vi "BoardUpdate.vi"(1 "Array":i32[][](array[numeric])=[[-3, -5, -4, -2, -1, -4, -5, -3], [-6, -6, -6, -6, -6, -6, -6, -6], [0, 0, 0, 0, 0, 0, 0, 0], [0, 0, 0, 0, 0, 0, 0, 0], [0, 0, 0, 0, 0, 0, 0, 0], [0, 0, 0, 0, 0, 0, 0, 0], [6, 6, 6, 6, 6, 6, 6, 6], [3, 5, 4, 2, 1, 4, 5, 3]], 2 "Clust Refnum":refnum<vi>) -> ()   [LabVIEW 2014]
doc: "Initialize cluster without array input, or update cluster with array input."
panel:
  in  "Colors [4]":cluster{u32, u32}[](array[cluster])=[{12369084, 12369084}, {9868950, 9868950}, {12369084, 12369084}, {9868950, 9868950}]
  out "Board 2":T1
  in  "Board":T1
  # "1:King\n2:Queen\n3:Rook\n4:Bishop\n5:Knight\n6:Pawn"
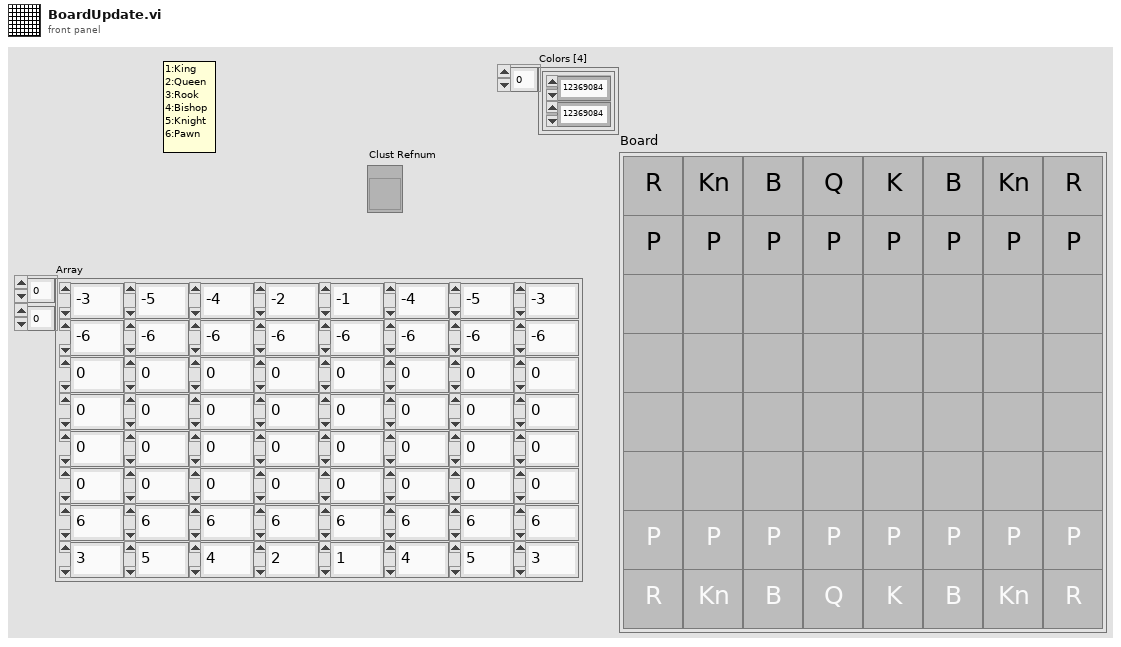
[diagram p1: front panel]
types:
  T1 = cluster{"OK Button 01":bool, "OK Button 02":bool, "OK Button 03":bool, "OK Button 04":bool, "OK Button 05":bool, "OK Button 06":bool, "OK Button 07":bool, "OK Button 08":bool, "OK Button 09":bool, "OK Button 10":bool, "OK Button 11":bool, "OK Button 12":bool, "OK Button 13":bool, "OK Button 14":bool, "OK Button 15":bool, "OK Button 16":bool, "OK Button 17":bool, "OK Button 18":bool, "OK Button 19":bool, "OK Button 20":bool, "OK Button 21":bool, "OK Button 22":bool, "OK Button 23":bool, "OK Button 24":bool, "OK Button 25":bool, "OK Button 26":bool, "OK Button 27":bool, "OK Button 28":bool, "OK Button 29":bool, "OK Button 30":bool, "OK Button 31":bool, "OK Button 32":bool, "OK Button 33":bool, "OK Button 34":bool, "OK Button 35":bool, "OK Button 36":bool, "OK Button 37":bool, "OK Button 38":bool, "OK Button 39":bool, "OK Button 40":bool, "OK Button 41":bool, "OK Button 42":bool, "OK Button 43":bool, "OK Button 44":bool, "OK Button 45":bool, "OK Button 46":bool, "OK Button 47":bool, "OK Button 48":bool, "OK Button 49":bool, "OK Button 50":bool, "OK Button 51":bool, "OK Button 52":bool, "OK Button 53":bool, "OK Button 54":bool, "OK Button 55":bool, "OK Button 56":bool, "OK Button 57":bool, "OK Button 58":bool, "OK Button 59":bool, "OK Button 60":bool, "OK Button 61":bool, "OK Button 62":bool, "OK Button 63":bool, "OK Button 64":bool}
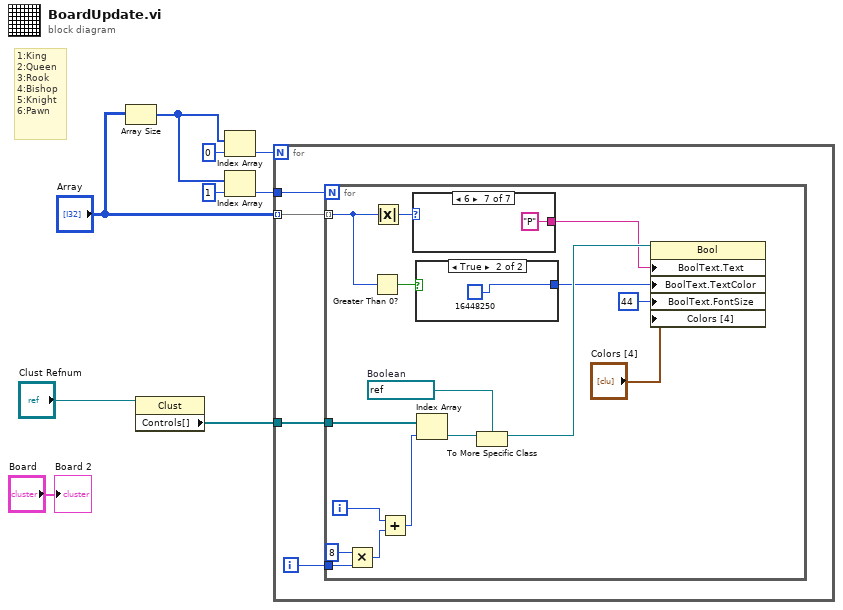
[diagram p0: block diagram]
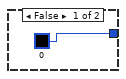
[diagram p2: hidden frame]
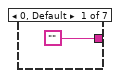
[diagram p3: hidden frame]
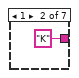
[diagram p4: hidden frame]
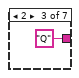
[diagram p5: hidden frame]
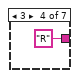
[diagram p6: hidden frame]
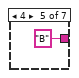
[diagram p7: hidden frame]
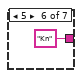
[diagram p8: hidden frame]
diagram:
  # "1:King\n2:Queen\n3:Rook\n4:Bishop\n5:Knight\n6:Pawn"
  n1 = Array Size(array="Array") -> (size(s)=w5:i32[])
  n2 = property class="Clust"(reference="Clust Refnum") -> ("Controls[]"=w3:refnum<vi>[])  [unwired: 1 in, 2 out]
  n3 = Index Array(array=w5, index=0) -> (element=w8:i32)
  n4 = Index Array(array=w5, index=1) -> (element=w4:i32)
  n5 = for {
    N: w8 -> [_]
    tunnel: "Array" -> [w12] mode=indexing
    tunnel: w4 -> [w13]
    tunnel: w3 -> [w11]
    i -> [w10]
    n6 = for {
      N: w13 -> [_]
      tunnel: w12 -> [w18] mode=indexing
      tunnel: w11 -> [w25]
      tunnel: w10 -> [w29]
      i -> [w27]
      w22 = refnum<vi> refnum  # Boolean
      n7 = Multiply(x=8, y=w29) -> (x*y=w26:i32)
      n8 = Greater Than 0?(x=w18) -> (x > 0?=w19:bool)
      n9 = Absolute Value(x=w18) -> (abs(x)=w20:i32)
      n10 = Add(x=w27, y=w26) -> (x+y=w24:i32)
      n11 = case shown="6" w20 {
        tunnel: ["" "K" "Q" "R" "B" "Kn" "P"] -> w16
        frame 0, Default {
        }
        frame 1 {
        }
        frame 2 {
        }
        frame 3 {
        }
        frame 4 {
        }
        frame 5 {
        }
        frame 6 {
        }
      }
      n12 = case shown="True" w19 {
        tunnel: [u32 0 u32 16448250] -> w17
        frame False {
        }
        frame True {
        }
      }
      n13 = Index Array(array=w25, index=w24) -> (element=w23:refnum<vi>)
      n14 = To More Specific Class(target class=w22, reference=w23) -> (specific class reference=w21:refnum<vi>)  [unwired: 1 in, 1 out]
      n15 = property class="Bool"(reference=w21, "BoolText.Text"=w16, "BoolText.TextColor"=w17, "BoolText.FontSize"=u32 44 ("Boolean Text.Font:Size"), "Colors [4]"="Colors [4]") -> ()  [unwired: 1 in, 2 out]
    }
  }
  "Board 2" <- "Board"
